vi "Listen.vi"(7 "Command Queue":refnum<class "Message Enqueuer.lvclass">, 8 "error in (no error)":errorcluster, 10 "Listen timeout ms":i32=100, 11 "Receiver in":refnum<class "Receiver.lvclass">) -> (0 "error out":errorcluster, 3 "Receiver out":refnum<class "Receiver.lvclass">)   [LabVIEW 2013, in "Receiver.lvlib" / "Receiver.lvclass"]
uses:
  Receiver.lvclass
  <vilib>/ActorFramework/Message Enqueuer/Message Enqueuer.lvclass
  Receiver.lvclass/Receiver.ctl
  <vilib>/ActorFramework/Message Enqueuer/Message Enqueuer.lvclass/Message Enqueuer.ctl
  <vilib>/ActorFramework/Message Enqueuer/Enqueue.vi
  <vilib>/ActorFramework/Message Priority Queue/Priority Enqueue.vi
  Receiver Command Messages/Listen Timeout Msg/Listen Timeout Msg.lvclass
panel:
  out "error out 3":errorcluster
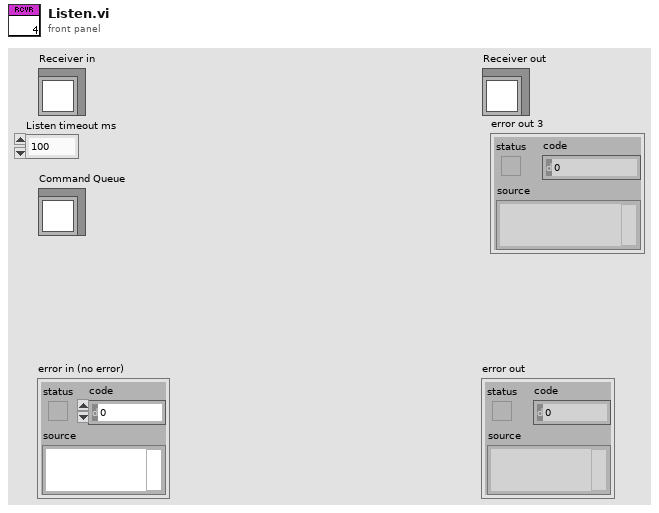
[diagram p1: front panel]
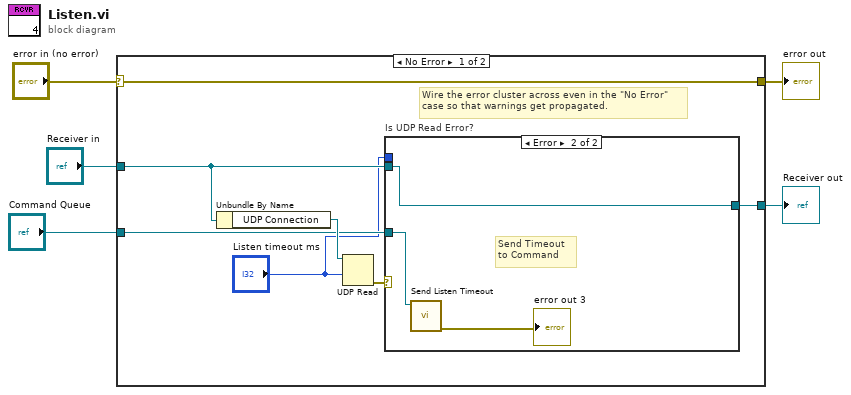
[diagram p0: block diagram]
diagram:
  n1 = case shown="No Error" "error in (no error)" {
    selector: "error in (no error)" -> [w12 w18]
    tunnel: [w12 w18] -> w4
    tunnel: [w8 w17] -> w2
    tunnel: "Receiver in" -> [w9 w17]
    tunnel: "Command Queue" -> [w7 _]
    frame No Error {
      # "Wire the error cluster across even in the \"No Error\"\ncase so that warnings get propagated."
      n2 = Unbundle By Name(w9) -> ("UDP Connection"=w11:refnum<k16>)
      n3 = UDP Read(connection ID=w11, timeout ms (25000)="Listen timeout ms") -> (error out=w10:errorcluster)  [unwired: 2 in, 4 out]
      n4 = case "Is UDP Read Error?" shown="Error" w10 {
        tunnel: w9 -> [w13 w16]
        tunnel: [w13 w16] -> w8
        tunnel: w7 -> [_ w15]
        tunnel: "Listen timeout ms" -> [_ _]
        frame No Error {
        }
        frame Error {
          # "Send Timeout \nto Command"
          n5 = call "Send Listen Timeout.vi"("Message Enqueuer"=w15) -> ("error out"=→"error out 3":errorcluster)  [unwired: 9 in, 1 out]
        }
      }
    }
    frame Error {
    }
  }
  "error out" <- w4
  "Receiver out" <- w2
